vi "Komm Modbus PMA.vi"() -> (0 "error IO":errorcluster)   [LabVIEW 2020, in "ABB-EL3000.lvlib" / "PMA.lvlib"]
uses:
  PMA.lvlib
  Allgemeine VI/Aktion FGV Modbus.ctl
  Stoerungen/Stoerungen Messgeraet/Aktionen Kommunikation Stoerung.ctl
  Allgemeine VI/Allgemeine VI.lvlib
  Stoerungen/Stoerungen.lvlib
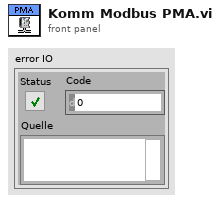
[diagram p1: front panel]
types:
  T1 = typedef "ABB-EL3000.lvlib/Allgemeine VI.lvlib/Aktion FGV Modbus.ctl" = enum16{"lesen", "Verbindung herstellen", "Verbindung trennen", "Komm", "Inaktiv"}
  T2 = typedef "Stoerungen.lvlib/Aktionen Kommunikation Stoerung.ctl" = enum16{"lesen", "init", "FT-IR Komm", "FT-IR Betriebsart", "FT-IR Hintergrund", "cRIO Komm", "PNS Komm", "Dichtheitstest", "Life Bit", "FTIR Komm AK", "PMA Komm", "FID Komm", "PMA Cal", "FID Ch4 Cal", "FID THC Cal", "Cal Timeout", "VFS 1 Komm", "VFS 2 Komm", "VFS 3 Komm", "VFS 4 Komm", "TRE 08 Komm", "CG-Test vorzeitig", "CG-Test Span 1", "CG-Test Span 2", "CG-Test Span 3", "CG-Test Messgas", "CG-Test löschen", "Test", "Amium AK", "AK Recept konfig", "AK Name konfig", "AK EKFG konfig"}
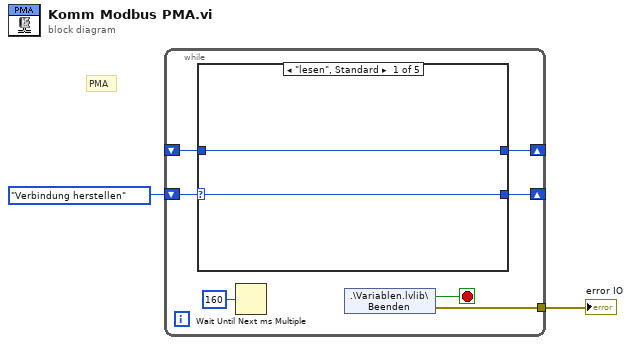
[diagram p0: block diagram]
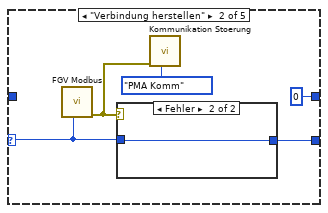
[diagram p2: hidden frame]
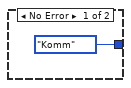
[diagram p3: hidden frame]
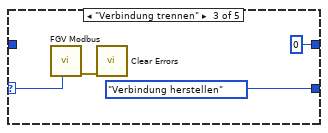
[diagram p4: hidden frame]
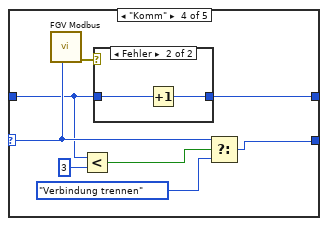
[diagram p5: hidden frame]
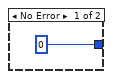
[diagram p6: hidden frame]
diagram:
  # "PMA"
  n1 = while {
    shift-right: [w9] -> _
    shift-left: Aktion_FGV_Modbus."Verbindung herstellen" ("Aktion") -> [w8]
    tunnel: [w5] -> w1
    shift-right: [w4] -> _
    shift-left: _ -> [w3]
    stop <- w6 stop-if-true
    n2 = case shown="\"lesen\", Standard" w8 {
      selector: w8 -> [w11 w14 w22 w29 w34]
      tunnel: [w11 w16 Aktion_FGV_Modbus."Verbindung herstellen" ("Aktion") w27 w34] -> w9
      tunnel: [w10 0 0 w26 w35] -> w4
      tunnel: w3 -> [w10 _ _ w25 w35]
      frame "lesen", Default {
      }
      frame "Verbindung herstellen" {
        n3 = call "FGV Modbus.vi"("Aktion"=w14) -> ("error out"=w12:errorcluster)  [unwired: 10 in]
        n4 = case shown="Fehler" w12 {
          tunnel: [Aktion_FGV_Modbus."Komm" ("Aktion") w18] -> w16
          tunnel: w14 -> [_ w18]
          frame No Error {
          }
          frame Error {
          }
        }
        n5 = call "Kommunikation Stoerung.vi"("Aktionen"=Aktionen_Kommunikation_Stoerung."PMA Komm", "error in"=w12) -> ()  [unwired: 9 in, 1 out]
      }
      frame "Verbindung trennen" {
        n6 = call "FGV Modbus.vi"("Aktion"=w22) -> ("error out"=w20:errorcluster)  [unwired: 10 in]
        n7 = call <vilib>:"Clear Errors.vi"("error in (no error)"=w20) -> ()  [unwired: 5 in, 2 out]
      }
      frame "Komm" {
        n8 = call "FGV Modbus.vi"("Aktion"=w29) -> ("error out"=w30:errorcluster)  [unwired: 10 in]
        n9 = Less?(x=w25, y=3) -> (x < y?=w23:bool)
        n10 = case shown="Fehler" w30 {
          tunnel: [0 w32] -> w26
          tunnel: w25 -> [_ w33]
          frame No Error {
          }
          frame Error {
            n11 = Increment(x=w33) -> (x+1=w32:i32)
          }
        }
        n12 = Select(t=w29, s=w23, f=Aktion_FGV_Modbus."Verbindung trennen" ("Aktion")) -> (s? t:f=w27:T1)
      }
      frame "Inaktiv" {
      }
    }
    n13 = Wait Until Next ms Multiple(millisecond multiple=u32 160 ("Vielfache von ms")) -> ()  [unwired: 1 out]
    n14 = shared-variable ".\\Variablen.lvlib\\Beenden"() -> (w6:bool, error out=w5:errorcluster)  [unwired: 1 in]
  }
  "error IO" <- w1
